vi "Enable.vi"(11 "logger in":refnum<class "Logger.lvclass">) -> (3 "logger out":refnum<class "Logger.lvclass">)   [LabVIEW 2018, in "Logging.lvlib" / "Logger.lvclass"]
uses:
  Logger.lvclass
  Logger.lvclass/Logger.ctl
  extension/scope_interface/Scope.lvclass
  extension/filter_interface/Filter.lvclass
  extension/formatting_handler_interface/Formatting Handler.lvclass
panel:
  # "Connector Pane"
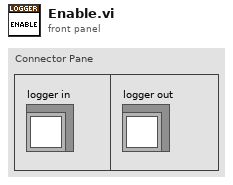
[diagram p1: front panel]
types:
  T1 = cluster{"Name":string, "Scope":string, "Filter":string, "Handler":string}
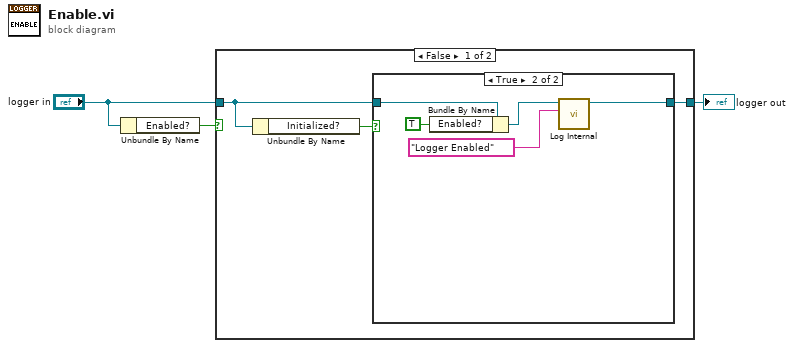
[diagram p0: block diagram]
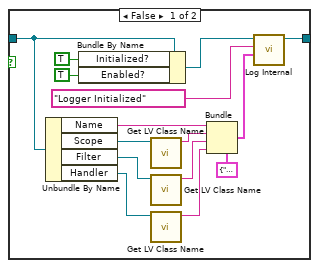
[diagram p2: hidden frame]
diagram:
  n1 = Unbundle By Name("logger in") -> ("Enabled?"=w2:bool)
  n2 = case shown="False" w2 {
    tunnel: "logger in" -> [w5 w27]
    tunnel: [w4 w27] -> w3
    frame False {
      n3 = Unbundle By Name(w5) -> ("Initialized?"=w6:bool)
      n4 = case shown="True" w6 {
        tunnel: w5 -> [w7 w26]
        tunnel: [w9 w25] -> w4
        frame False {
          n5 = Unbundle By Name(w7) -> ("Name"=w16:string, "Scope"=w20:refnum<class "Scope.lvclass">, "Filter"=w19:refnum<class "Filter.lvclass">, "Handler"=w18:refnum<class "Formatting Handler.lvclass">)
          n6 = Bundle By Name(cluster=w7, "Initialized?"=TRUE, "Enabled?"=TRUE) -> (w8:refnum<class "Logger.lvclass">)
          n7 = call <vilib>:"Get LV Class Name.vi"("object"=w20) -> ("class name"=w17:string)  [unwired: 9 in, 1 out]
          n8 = call <vilib>:"Get LV Class Name.vi"("object"=w19) -> ("class name"=w15:string)  [unwired: 9 in, 1 out]
          n9 = call <vilib>:"Get LV Class Name.vi"("object"=w18) -> ("class name"=w14:string)  [unwired: 9 in, 1 out]
          n10 = Bundle(cluster=T1 {"Name"="", "Scope"="", "Filter"="", "Handler"=""}, "Name"=w16, "Scope"=w17, "Filter"=w15, "Handler"=w14) -> (w12:T1)
          n11 = call "Log Internal.vi"("data (null)"=w12, "message"="Logger Initialized", "logger in"=w8) -> ("logger out"=w9:refnum<class "Logger.lvclass">)  [unwired: 8 in]
        }
        frame True {
          n12 = Bundle By Name(cluster=w26, "Enabled?"=TRUE) -> (w23:refnum<class "Logger.lvclass">)
          n13 = call "Log Internal.vi"("message"="Logger Enabled", "logger in"=w23) -> ("logger out"=w25:refnum<class "Logger.lvclass">)  [unwired: 9 in]
        }
      }
    }
    frame True {
    }
  }
  "logger out" <- w3
